vi "fg_indicator.vi"(8 "Mode selector":T1=enum."GET", 11 "Numeric":dbl) -> (1 "time at restart":timestamp, 2 "Time since reset":dbl, 3 "Output":dbl)   [LabVIEW 2022 SP3]
uses:
  fg_enum.ctl
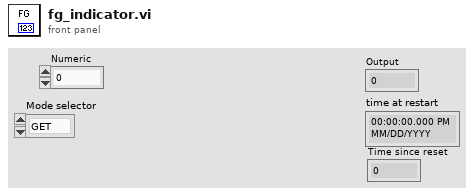
[diagram p1: front panel]
types:
  T1 = typedef "fg_enum.ctl" = enum16{"SET", "RESET TIME", "GET"}
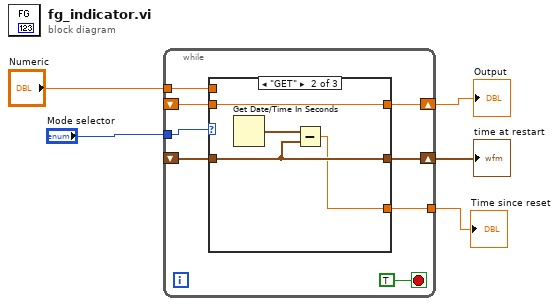
[diagram p0: block diagram]
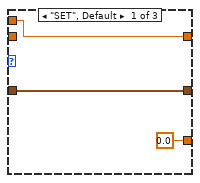
[diagram p2: hidden frame]
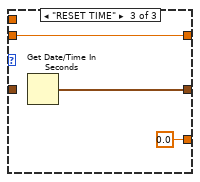
[diagram p3: hidden frame]
diagram:
  n1 = while {
    tunnel: "Mode selector" -> [w12]
    shift-right: [w10] -> w1
    shift-left: _ -> [w11]
    tunnel: "Numeric" -> [w9]
    shift-right: [w8] -> w4
    shift-left: _ -> [w7]
    tunnel: [w6] -> w3
    stop <- TRUE stop-if-true
    n2 = case shown="\"GET\"" w12 {
      tunnel: w11 -> [_ w20 w22]
      tunnel: [w15 w20 w22] -> w10
      tunnel: w9 -> [w15 _ _]
      tunnel: [w16 w18 w23] -> w8
      tunnel: w7 -> [w16 w18 _]
      tunnel: [0.0 w17 0.0] -> w6
      frame "SET", Default {
      }
      frame "GET" {
        n3 = Get Date/Time In Seconds() -> (seconds since 1Jan1904=w19:timestamp)
        n4 = Subtract(x=w19, y=w18) -> (x-y=w17:dbl)
      }
      frame "RESET TIME" {
        n5 = Get Date/Time In Seconds() -> (seconds since 1Jan1904=w23:timestamp)
      }
    }
  }
  "time at restart" <- w4
  "Time since reset" <- w3
  "Output" <- w1
